vi "rtout_setTriggerConfig.vi"(0 "connection ID":refnum<k5>, 1 "axis":i32, 2 "higher":i32, 3 "lower":i32, 4 "epsilon":i32, 5 "error":errorcluster, 6 "polarity":i32) -> (14 "connection ID out":refnum<k5>, 15 "axis_out":i32, 19 "error out":errorcluster)   [LabVIEW 2016, in "amc_api.lvlib"]
doc: "Control the real time output trigger config"
uses:
  amc_api.lvlib
panel:
  out "jsonRespIn":string
  out "JSON-response":string="{\"jsonrpc\":\"2.0\",\"method\":\"\",\"params\":[5,1.245,true,\"name\"],\"id\":\"1\"}"
  out "JSON request":string
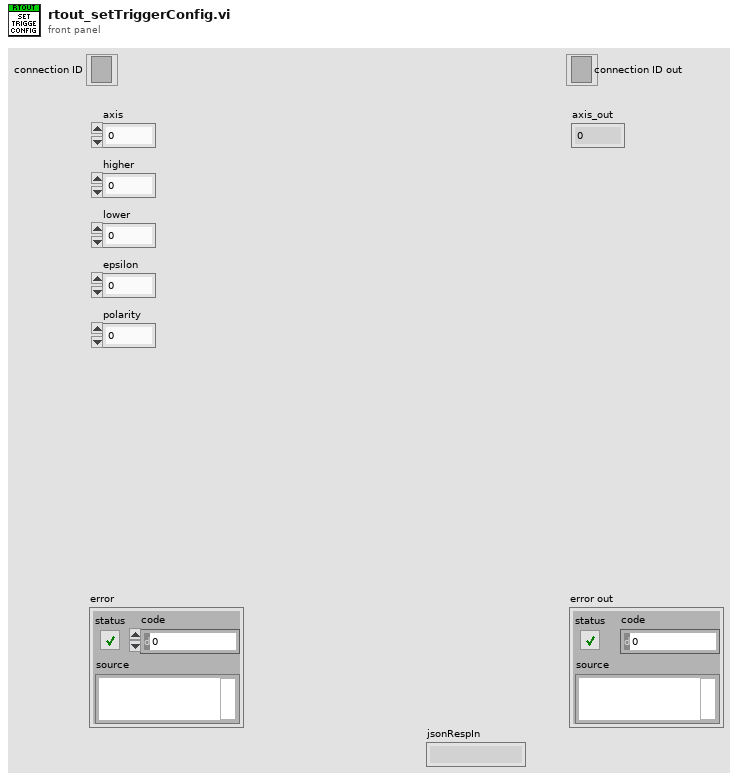
[diagram p1: front panel]
types:
  T1 = cluster{"jsonrpc":string, "method":string, "params":string[], "id":string, "api":i32, "pid":string}
  T2 = enum16{"Standard", "Buffered", "CRLF", "Immediate"}
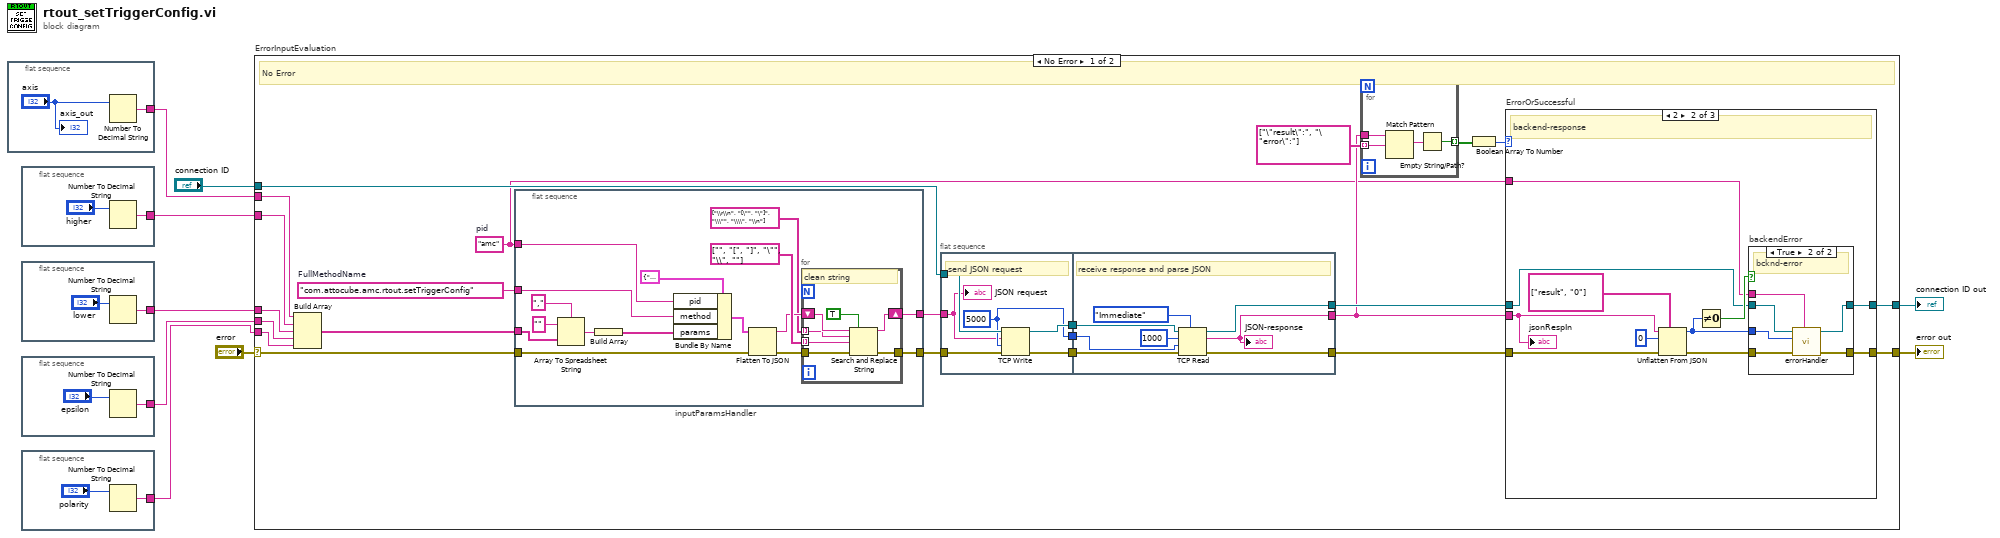
[diagram p0: block diagram]
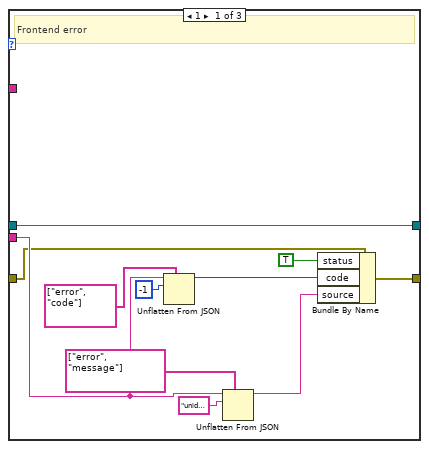
[diagram p2: hidden frame]
diagram:
  n1 = flat-sequence "in_axis" {
    tunnel: [w11] -> w5
    frame #0 {
      n2 = Number To Decimal String(number="axis") -> (decimal integer string=w11:string)  [unwired: 1 in]
      "axis_out" <- "axis"
    }
  }
  n3 = flat-sequence "in_integer" {
    tunnel: [w12] -> w4
    frame #0 {
      n4 = Number To Decimal String(number="higher") -> (decimal integer string=w12:string)  [unwired: 1 in]
    }
  }
  n5 = flat-sequence "in_integer" {
    tunnel: [w14] -> w3
    frame #0 {
      n6 = Number To Decimal String(number="lower") -> (decimal integer string=w14:string)  [unwired: 1 in]
    }
  }
  n7 = flat-sequence "in_integer" {
    tunnel: [w16] -> w2
    frame #0 {
      n8 = Number To Decimal String(number="epsilon") -> (decimal integer string=w16:string)  [unwired: 1 in]
    }
  }
  n9 = flat-sequence "in_integer" {
    tunnel: [w18] -> w1
    frame #0 {
      n10 = Number To Decimal String(number="polarity") -> (decimal integer string=w18:string)  [unwired: 1 in]
    }
  }
  n11 = case "ErrorInputEvaluation" shown="No Error" "error" {
    selector: "error" -> [w35 w116]
    tunnel: "connection ID" -> [w39 w117]
    tunnel: [w26 w116] -> w8
    tunnel: [w27 w117] -> w7
    tunnel: w5 -> [w24 _]
    tunnel: w4 -> [w23 _]
    tunnel: w3 -> [w22 _]
    tunnel: w2 -> [w21 _]
    tunnel: w1 -> [w20 _]
    frame No Error {
      w25 = "amc"  # pid
      w36 = "com.attocube.amc.rtout.setTriggerConfig"  # FullMethodName
      # "No Error"
      n12 = Build Array ("ParametersArrayString")(w24, w23, w22, w21, w20) -> (w34:string[])
      n13 = flat-sequence "inputParamsHandler" {
        tunnel: [w80] -> w33
        tunnel: w34 -> [w86]
        tunnel: w35 -> [w85]
        tunnel: [w82] -> w32
        tunnel: w36 -> [w76]
        tunnel: w25 -> [w75]
        frame #0 {
          n14 = Array To Spreadsheet String(delimiter (Tab)=",", array=w86, 3:"" ("format string")) -> (spreadsheet string=w88:string)
          n15 = Build Array "Build Array"(w88) -> (w77:string[])
          n16 = Bundle By Name(cluster=T1 {"jsonrpc"="2.0", "method"="com.attocube.amc.res.setRESReadOutFreq", "params"=[], "id"="1", "api"=2, "pid"=""} ("Cluster"), "pid"=w75, "method"=w76, "params"=w77) -> (w87:T1)
          n17 = Flatten To JSON(anything=w87, error in (no error)=w85) -> (JSON string=w81:string, 11:w83:errorcluster)  [unwired: 1 in]
          n18 = for {
            tunnel: string[] ["\\r\\n", "[\"", "\"]", "\\\"", "\\\\", "\\n"] ("search string") -> [w94] mode=indexing
            tunnel: string[] ["", "[", "]", "\"", "\\", ""] ("replace string (\"\")") -> [w93] mode=indexing
            shift-right: [w96] -> w80
            shift-left: w81 -> [w95]
            tunnel: w83 -> [w92]
            tunnel: [w91] -> w82
            # "clean string"
            n19 = Search and Replace String(replace all?=TRUE ("replace all? (F)"), input string=w95, search string=w94, replace string=w93, error in=w92) -> (result string=w96:string, error out=w91:errorcluster)  [unwired: 3 in, 2 out]
          }
        }
      }
      n20 = flat-sequence {
        tunnel: w39 -> [w107]
        tunnel: [w105] -> w42
        tunnel: [w106] -> w41
        tunnel: w32 -> [w102]
        tunnel: [w104] -> w40
        tunnel: w33 -> [w103]
        tunnel: [w111] -> w31
        tunnel: w42 -> [w113]
        tunnel: w41 -> [w112]
        tunnel: [w109] -> w30
        tunnel: w40 -> [w110]
        tunnel: [w108] -> w29
        frame #0 {
          w104 = 5000 ("timeout ms (25000)")
          # "send JSON request"
          n21 = TCP Write(connection ID=w107, data in=w103, error in (no error)=w102, 9:w104) -> (connection ID out=w105:refnum<k5>, error out=w106:errorcluster)  [unwired: 1 out]
          "JSON request" <- w103
        }
        frame #1 {
          # "receive response and parse JSON"
          n22 = TCP Read(connection ID=w113, bytes to read=1000, error in (no error)=w112, 7:T2."Immediate" ("mode (standard)"), 9:w110) -> (connection ID out=w111:refnum<k5>, data out=w108:string, error out=w109:errorcluster)
          "JSON-response" <- w108
        }
      }
      n23 = for {
        tunnel: string[] ["\"result\":", "\"error\":"] ("path") -> [w100] mode=indexing
        tunnel: [w98] -> w37 mode=indexing
        tunnel: w29 -> [w101]
        n24 = Match Pattern(string=w101, regular expression=w100) -> (match substring=w99:string)  [unwired: 1 in, 3 out]
        n25 = Empty String/Path?(string/path=w99) -> (empty?=w98:bool)
      }
      n26 = Boolean Array To Number(Boolean array=w37) -> (number=w28:u32)
      n27 = case "ErrorOrSuccessful" shown="2" w28 {
        tunnel: w29 -> [w45 w56 _]
        tunnel: w31 -> [w43 w58 w74]
        tunnel: [w43 w57 w74] -> w27
        tunnel: [w46 w54 w73] -> w26
        tunnel: w30 -> [w44 w55 w73]
        tunnel: w25 -> [_ w59 _]
        frame 1 {
          # "Frontend error"
          n28 = Unflatten From JSON(path=string[] ["error", "code"], JSON string=w45, type and defaults=-1) -> (value=w52:i32)  [unwired: 4 in, 1 out]
          n29 = Unflatten From JSON(path=string[] ["error", "message"], JSON string=w45, type and defaults="unidentified error") -> (value=w53:string)  [unwired: 4 in, 1 out]
          n30 = Bundle By Name(cluster=w44, "status"=TRUE, "code"=w52, "source"=w53) -> (w46:errorcluster)
        }
        frame 2 {
          # "backend-response"
          n31 = Unflatten From JSON(path=string[] ["result", "0"], JSON string=w56, type and defaults=0, error in (no error)=w55) -> (value=w60:i32, error out=w62:errorcluster)  [unwired: 3 in]
          n32 = Not Equal To 0?(x=w60) -> (x != 0?=w61:bool)
          n33 = case "backendError" shown="True" w61 {
            tunnel: w60 -> [_ w72]
            tunnel: w62 -> [w66 w71]
            tunnel: [w65 w70] -> w57
            tunnel: [w66 w69] -> w54
            tunnel: w58 -> [w65 w68]
            tunnel: w59 -> [_ w67]
            frame False {
              # "successful"
            }
            frame True {
              # "bcknd-error"
              n34 = call "errorHandler.vi"("pid"=w67, "error in"=w71, "errNbr"=w72, "connection ID"=w68) -> ("error out 2"=w69:errorcluster, "connection ID out"=w70:refnum<k5>)  [unwired: 6 in]
            }
          }
          "jsonRespIn" <- w56
        }
        frame Default {
          # "NoResponse"
        }
      }
    }
    frame Error {
      # "Error"
    }
  }
  "error out" <- w8
  "connection ID out" <- w7
